vi "Get Attribute STRING.vi"(8 "error in":errorcluster, 10 "Attribute":string, 11 "Config from XML in":refnum<class "Config from XML.lvclass">) -> (0 "error out":errorcluster, 2 "Value":string, 3 "Config from XML out":refnum<class "Config from XML.lvclass">)   [LabVIEW 2024, in "Config from XML.lvclass"]
uses:
  Config from XML.lvclass
  Config from XML.lvclass/Config from XML.ctl
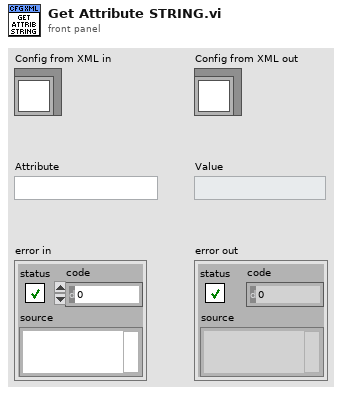
[diagram p1: front panel]
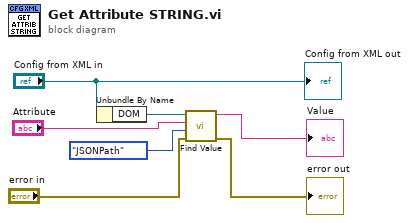
[diagram p0: block diagram]
diagram:
  n1 = Unbundle By Name("Config from XML in") -> ("DOM"=w2:refnum<k20>)
  n2 = call "Find Value.vi"("error in"="error in", "Path Style"=enum16{"JSONPath", "XPath"}."JSONPath", "Attribute"="Attribute", "DOM"=w2) -> ("error out"=→"error out":errorcluster, "Value"=→"Value":string)  [unwired: 6 in]
  "Config from XML out" <- "Config from XML in"
